vi "predict.vi"(8 "error in (no error)":errorcluster, 11 "Interface_predict_with_std in":refnum<class "Interface_predict_with_std.lvclass">) -> (0 "error out":errorcluster, 2 "out":cluster{"y_mean":dbl[], "y_std":dbl[]}, 3 "Interface_predict_with_std out":refnum<class "Interface_predict_with_std.lvclass">)   [LabVIEW 2020, in "Interface_predict_with_std.lvclass"]
doc: "Predict using the linear model.\n\nIn addition to the mean of the predictive distribution, also its standard deviation can be returned."
uses:
  Interface_predict_with_std.lvclass
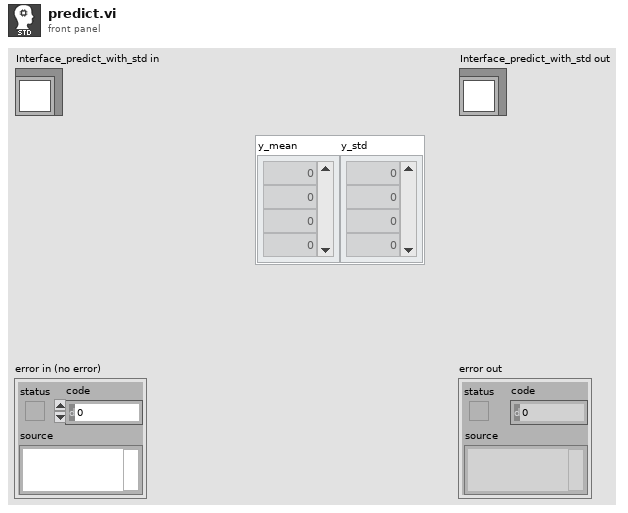
[diagram p1: front panel]
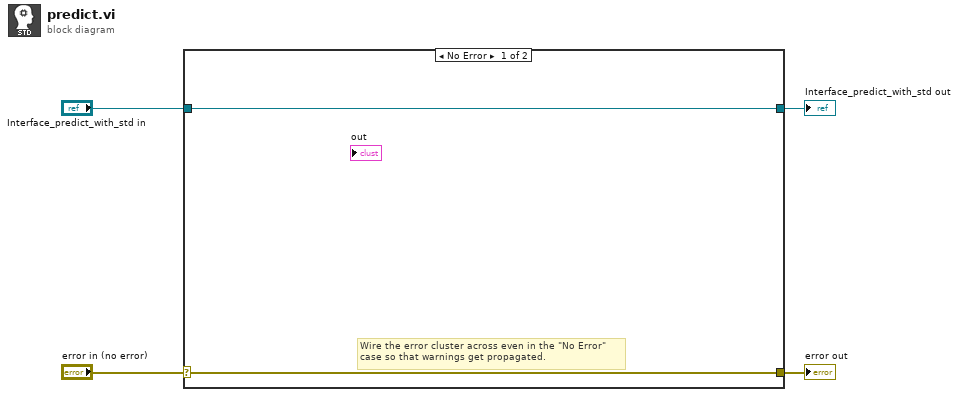
[diagram p0: block diagram]
diagram:
  n1 = case shown="No Error" "error in (no error)" {
    selector: "error in (no error)" -> [w5 w8]
    tunnel: [w5 w8] -> w3
    tunnel: [w6 w7] -> w1
    tunnel: "Interface_predict_with_std in" -> [w6 w7]
    frame No Error {
      # "Wire the error cluster across even in the \"No Error\"\ncase so that warnings get propagated."
    }
    frame Error {
    }
  }
  "error out" <- w3
  "Interface_predict_with_std out" <- w1
